vi "VCS Set Ec Motor Parameter.vi"(0 "axis in":cluster{"keyHandle":u32, "nodeId":u16}={"keyHandle"=0, "nodeId"=1}, 5 "EC motor parameter":T1, 11 "error in (no error)":errorcluster) -> (4 "axis out":cluster{"keyHandle":u32, "nodeId":u16}={"keyHandle"=0, "nodeId"=1}, 15 "error out":errorcluster)   [LabVIEW 2018]
doc: "With function <B>VCS_SetEcMotorParameter</B> it is possible to write all EC motor parameters."
uses:
  Resources/EposCmd.dll
  Resources/EposCmd64.dll
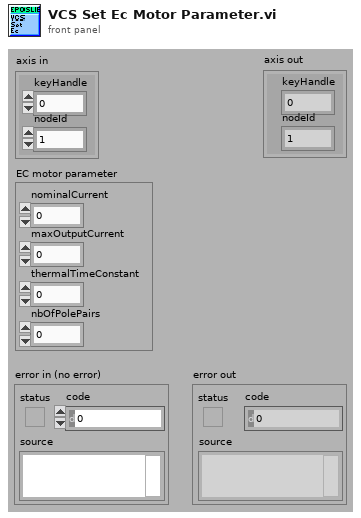
[diagram p1: front panel]
types:
  T1 = cluster{"nominalCurrent":u16, "maxOutputCurrent":u16, "thermalTimeConstant":u16, "nbOfPolePairs":u8}
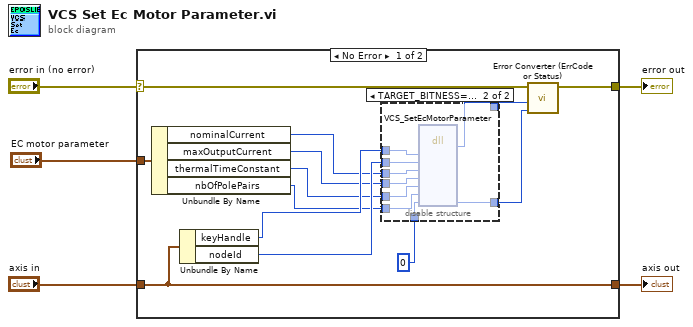
[diagram p0: block diagram]
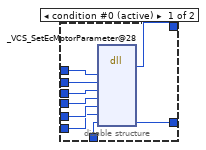
[diagram p2: hidden frame]
diagram:
  n1 = case shown="No Error" "error in (no error)" {
    selector: "error in (no error)" -> [w16 w37]
    tunnel: "axis in" -> [w18 w38]
    tunnel: [w18 w38] -> w4
    tunnel: [w17 w37] -> w3
    tunnel: "EC motor parameter" -> [w10 _]
    frame No Error {
      n2 = Unbundle By Name(w10) -> ("nominalCurrent"=w9:u16, "maxOutputCurrent"=w8:u16, "thermalTimeConstant"=w7:u16, "nbOfPolePairs"=w6:u8)
      n3 = Unbundle By Name(w18) -> ("keyHandle"=w11:u32, "nodeId"=w12:u16)
      n4 = disable-structure shown="TARGET_BITNESS==64" {
        disable-tunnel: [w27 w36] -> w15
        disable-tunnel: [w26 w35] -> w14
        disable-tunnel: u32 0 ("pErrorCode") -> [w25 w34]
        disable-tunnel: w12 -> [w24 w33]
        disable-tunnel: w11 -> [w23 w32]
        disable-tunnel: w9 -> [w22 w31]
        disable-tunnel: w8 -> [w21 w30]
        disable-tunnel: w7 -> [w20 w29]
        disable-tunnel: w6 -> [w19 w28]
        frame condition #0 (active) {
          n5 = dll-call lib="C:/Projeto em LabVIEW/EPOS-LabVIEW-Instrument-Driver-En/LabVIEW/maxon EPOS/Resources/EposCmd.*" fn="_VCS_SetEcMotorParameter@28"("KeyHandle"=w23, "NodeId"=w24, "NominalCurrent"=w22, "MaxOutputCurrent"=w21, "ThermalTimeConstant"=w20, "NbOfPolePairs"=w19, "pErrorCode"=w25) -> (w27:i32, "pErrorCode"=w26:u32)  [unwired: 9 in, 2 out]
        }
        frame condition #1 {
          n6 = dll-call lib="C:/setup/Resources/EposCmd64.*" fn="VCS_SetEcMotorParameter" ("EposCmd.dll:_VCS_SetEcMotorParameter@28")("KeyHandle"=w32, "NodeId"=w33, "NominalCurrent"=w31, "MaxOutputCurrent"=w30, "ThermalTimeConstant"=w29, "NbOfPolePairs"=w28, "pErrorCode"=w34) -> ("Rückgabetyp"=w36:i32, "pErrorCode"=w35:u32)  [unwired: 9 in, 2 out]
        }
      }
      n7 = call "Error Converter (ErrCode or Status).vi"("error code"=w14, "return type"=w15, "error in (no error)"=w16) -> ("error out"=w17:errorcluster)  [unwired: 7 in]
    }
    frame Error {
    }
  }
  "error out" <- w3
  "axis out" <- w4
